vi "endianness test.vi"() -> ()   [LabVIEW 2013, in "Profibus Module tests.lvlib"]
uses:
  Profibus Module tests.lvlib
  execution/profibus slave configuration.ctl
  execution/profibus mapping configuration.ctl
  <vilib>/NI/Tag Bus/tag/Data Type.ctl
  configuration/Profibus Module configuration.lvclass
  configuration/endianness setting.ctl
  channel/Profibus channel.lvclass
  <vilib>/NI/Tag Bus Module Framework/channel/channel classification.ctl
  channel/Profibus channel.lvclass/Profibus channel.ctl
  <vilib>/NI/Tag Bus Module Framework/channel/TBM channel.lvclass/TBM channel.ctl
  <vilib>/NI/Tag Bus/tag/tag descriptor.lvclass/tag descriptor.ctl
  configuration/Profibus Module configuration.lvclass/Profibus Module configuration.ctl
  channel/Write slave.vi
  channel/Write byte.vi
  <vilib>/NI/Tag Bus Module Framework/channel/Write channel classification.vi
  <vilib>/NI/Tag Bus/tag/write data type.vi
  <vilib>/NI/Tag Bus/tag/write tag name.vi
  <vilib>/NI/Tag Bus/table/data polymorphs/write one/write U8.vi
  <vilib>/NI/Tag Bus/table/data polymorphs/write one/write U16.vi
  <vilib>/NI/Tag Bus/table/data polymorphs/write one/write U32.vi
  configuration/Write byte orders.vi
  configuration/Read profibus channels.vi
  execution/calculate last byte.vi
  <vilib>/NI/Tag Bus/tag/read tag name.vi
  <vilib>/NI/Tag Bus/tag/read data type.vi
  <vilib>/NI/Tag Bus Module Framework/channel/Read channel classification.vi
  channel/Read slave.vi
  channel/Read byte.vi
  channel/Read bit.vi
  configuration/Read byte orders.vi
  execution/set endianness.vi
  <vilib>/NI/Tag Bus/dictionary/locate tag.vi
  execution/slave not available error.vi
  execution/data out of range.vi
  <vilib>/NI/Tag Bus/dictionary/data dictionary.lvclass
  <vilib>/NI/Tag Bus Module Framework/channel/TBM channel.lvclass
  <vilib>/NI/Tag Bus Module Framework/runtime/TBM module execution interface.lvclass
  execution/Profibus Module runtime.lvclass
  <vilib>/NI/Tag Bus Module Framework/root configuration/TBM configuration.lvclass
  <vilib>/NI/Tag Bus/tag/tag descriptor.lvclass
  <vilib>/NI/Tag Bus/table/data table.lvlib
panel:
  out "in":cluster{"U32":u32, "U16":u16, "U8":u8}[](array[cluster])
  out "16b":u16
  out "16l":u16
  out "32b":u32
  out "32l":u32
  out "u32b":u8[](array[numeric])
  out "u16b":u8[](array[numeric])
  out "out":u8[][](array[numeric])
  out "outputs":T1[](array[typedef])
  out "inputs":T1[](array[typedef])
  out "error out":errorcluster
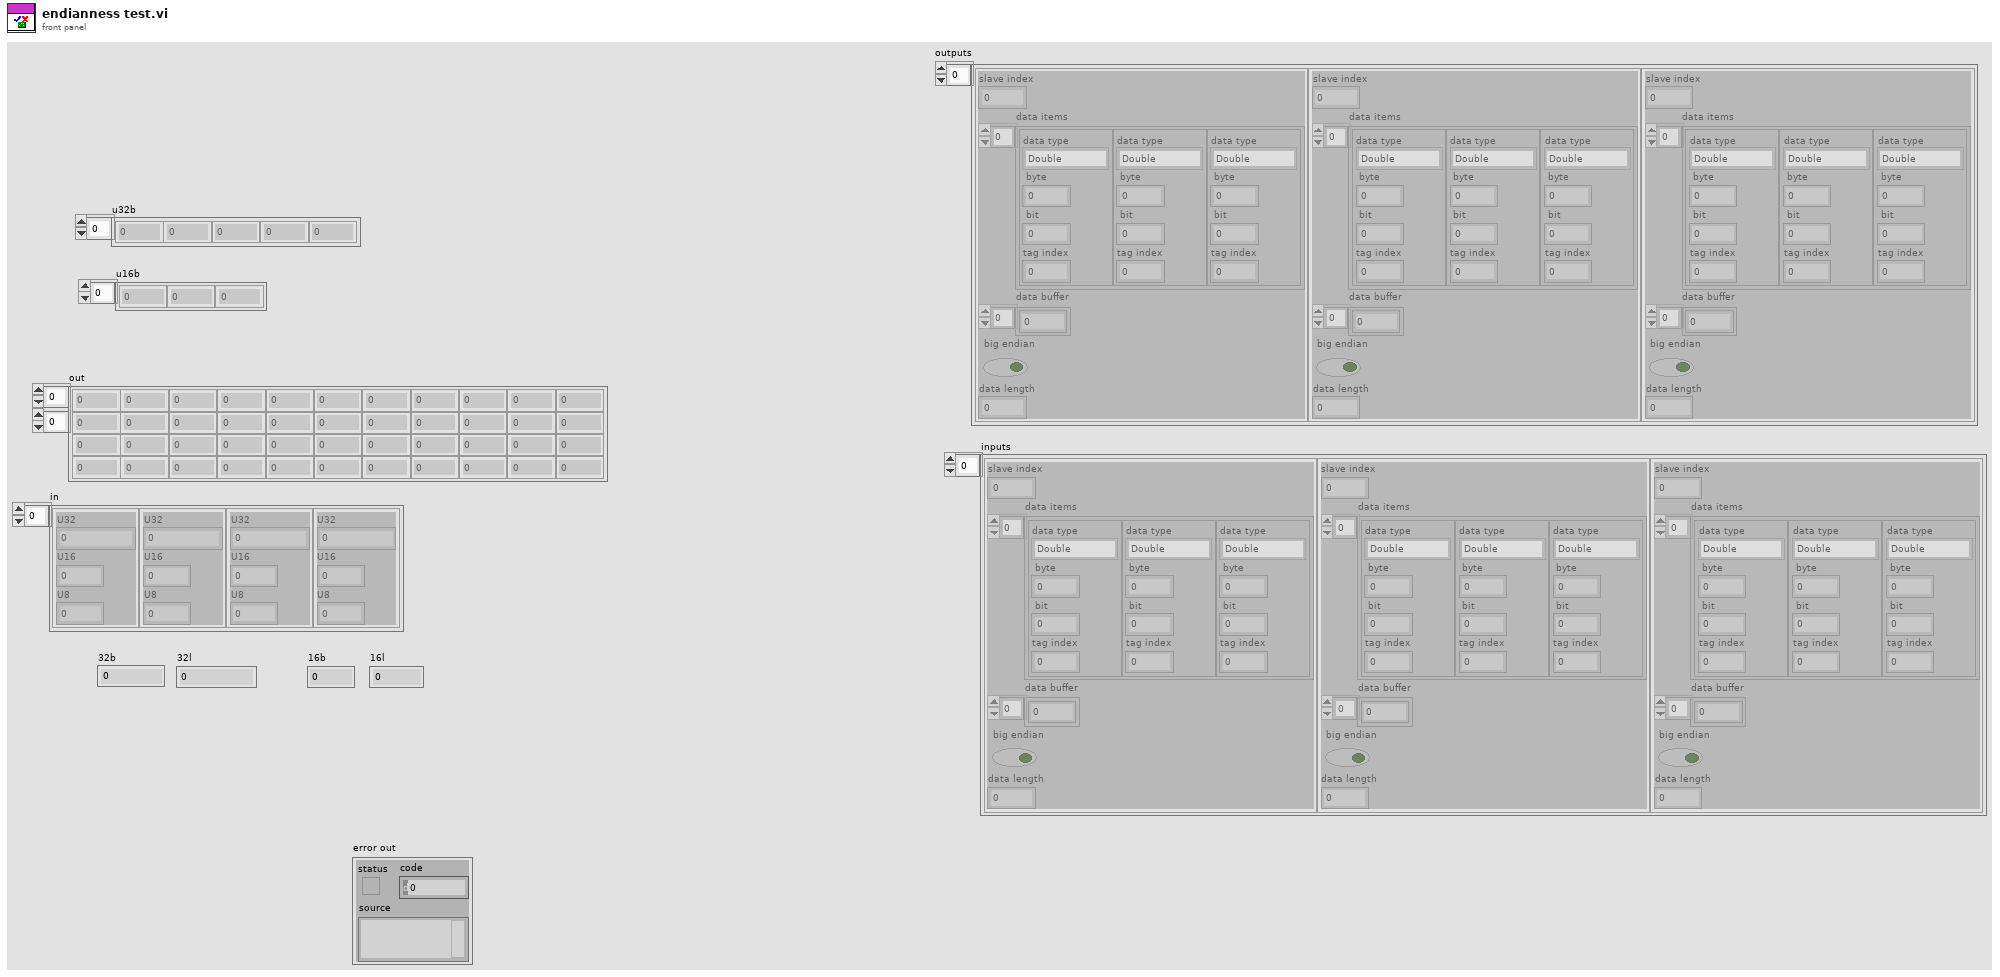
[diagram p1: front panel]
types:
  T1 = typedef "Profibus Module runtime.lvclass/profibus slave configuration.ctl" = cluster{"slave index":i8, "data items":T2[], "data buffer":u8[], "big endian":bool, "data length":i32}
  T2 = typedef "Profibus Module runtime.lvclass/profibus mapping configuration.ctl" = cluster{"data type":T3, " byte":i32, " bit":i32, "tag index":i32}
  T3 = typedef "tag bus.lvlib/tag descriptor.lvclass/Data Type.ctl" = enum16{"Double", "Single", "I64", "I32", "I16", "I8", "U64", "U32", "U16", "U8", "Boolean", "String", "Array of Double", "Array of Single", "Array of I64", "Array of I32", "Array of I16", "Array of I8", "Array of U64", "Array of U32", "Array of U16", "Array of U8", "Array of Boolean", "Array of String"}
  T4 = typedef "TBM channel.lvclass/channel classification.ctl" = enum16{"input data", "output data", "processing parameter", "processing result"}
  T5 = cluster{"Address":i8, "Input Length":u8, "Output Length":u8}[]
  T6 = typedef "Profibus Module configuration.lvclass/endianness setting.ctl" = cluster{"slave":i8, "big endian":bool}
  T7 = typedef "TBM channel.lvclass/data tables.ctl" = cluster{"input data":T8, "processing parameter":T8, "processing result":T8, "output data":T8}
  T8 = typedef "tag bus.lvlib/dictionary table pair.ctl" = cluster{"data dictionary":refnum<class "data dictionary.lvclass">, "data table":T9}
  T9 = typedef "tag bus.lvlib/data table.lvlib/data table.ctl" = cluster{"Double":dbl[], "Single":sgl[], "I64":i64[], "I32":i32[], "I16":i16[], "I8":i8[], "U64":u64[], "U32":u32[], "U16":u16[], "U8":u8[], "Boolean":bool[], "String":string[], "Array of Double":cluster{"DBL Array":dbl[]}[], "Array of Single":cluster{"SGL Array":sgl[]}[], "Array of I64":cluster{"I64 Array":i64[]}[], "Array of I32":cluster{"I32 Array":i32[]}[], "Array of I16":cluster{"I16 Array":i16[]}[], "Array of I8":cluster{"I8 Array":i8[]}[], "Array of U64":cluster{"U64 Array":u64[]}[], "Array of U32":cluster{"U32 Array":u32[]}[], "Array of U16":cluster{"U16 Array":u16[]}[], "Array of U8":cluster{"U8 Array":u8[]}[], "Array of Boolean":cluster{"Boolean Array":bool[]}[], "Array of String":cluster{"String Array":string[]}[]}
  T10 = typedef "TBM module execution interface.lvclass/execution settings.ctl" = cluster{"reads inputs":bool, "processes data":bool, "writes outputs":bool}
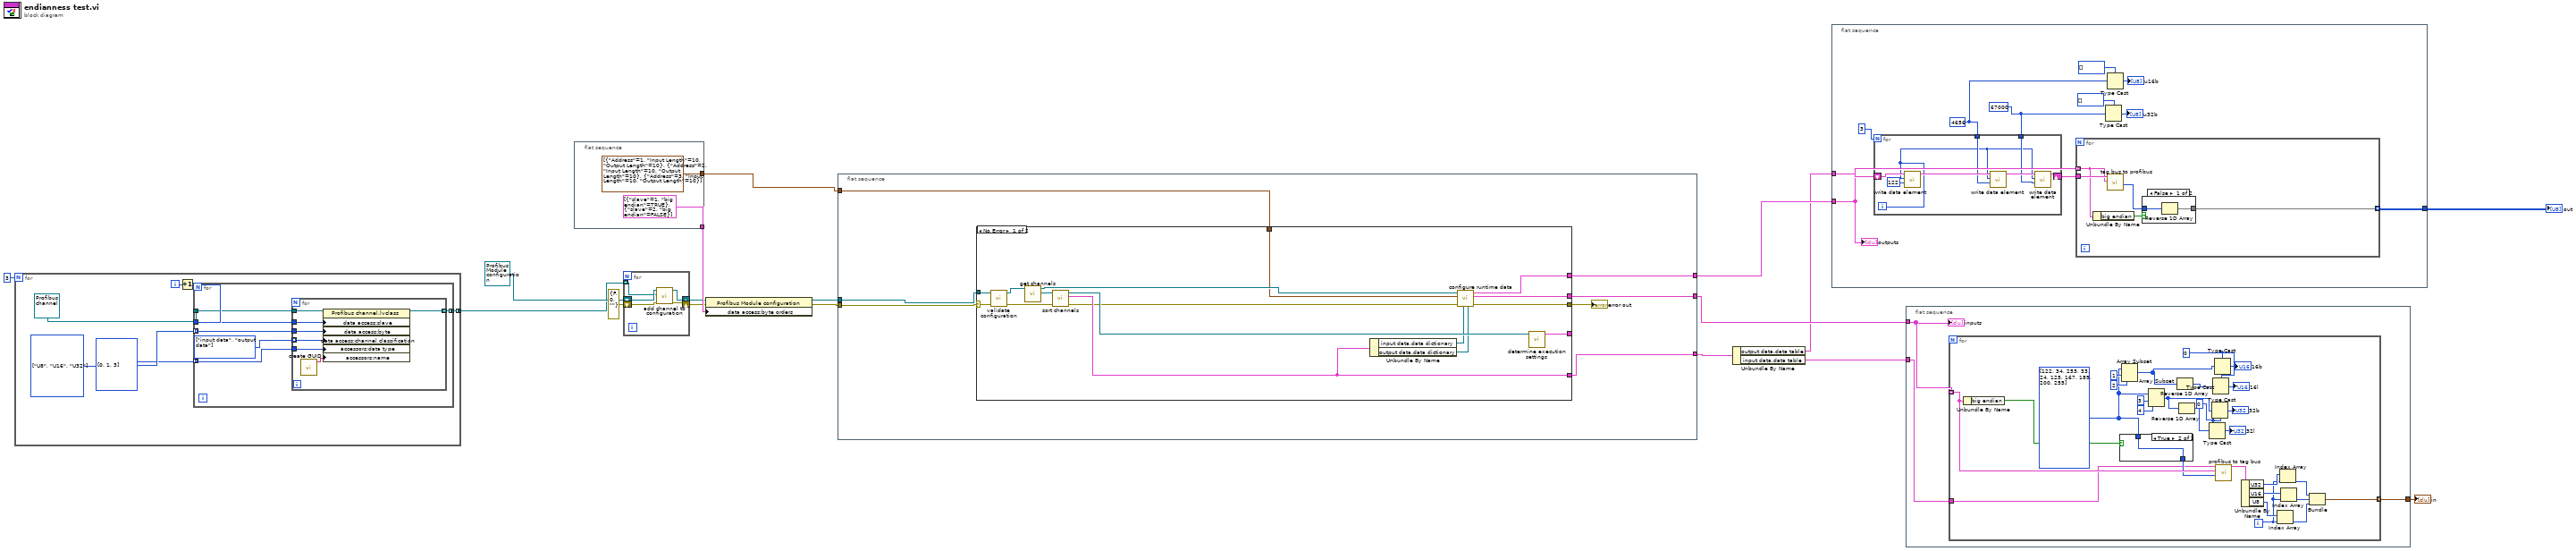
[diagram p0: block diagram]
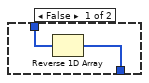
[diagram p2: hidden frame]
diagram:
  n1 = for {
    N: 3 -> [_]
    tunnel: [w22] -> w9 mode=concatenating
    i -> [w21]
    w18 = T3[] [enum."U8", enum."U16", enum."U32"] items=["Double", "Single", "I64", "I32", "I16", "I8", "U64", "U32", "U16", "U8", "Boolean", "String", "Array of Double", "Array of Single", "Array of I64", "Array of I32", "Array of I16", "Array of I8", "Array of U64", "Array of U32", "Array of U16", "Array of U8", "Array of Boolean", "Array of String"]
    n2 = Increment(x=w21) -> (x+1=w20:i32)
    n3 = for {
      tunnel: refnum<class "Profibus channel.lvclass"> refnum ("Profibus channel.lvclass") -> [w29]
      tunnel: [w28] -> w22 mode=concatenating
      tunnel: w20 -> [w27]
      tunnel: i32[] [0, 1, 3] -> [w25] mode=indexing
      tunnel: w18 -> [w24] mode=indexing
      w26 = T4[] [enum."input data", enum."output data"] items=["input data", "output data", "processing parameter", "processing result"]
      n4 = for {
        tunnel: w29 -> [w36]
        tunnel: [w35] -> w28 mode=indexing
        tunnel: w27 -> [w34]
        tunnel: w26 -> [w32] mode=indexing
        tunnel: w25 -> [w31]
        tunnel: w24 -> [w30]
        n5 = call <vilib>:"create GUID.vi"() -> ("uuid"=w33:string)  [unwired: 11 in]
        n6 = property class="Profibus channel.lvclass"(reference=w36, "data access:slave"=w34, "data access:byte"=w31, "data access:channel classification"=w32, "accessors:data type"=w30, "accessors:name"=w33) -> (reference out=w35:refnum<class "Profibus channel.lvclass">)  [unwired: 1 in, 1 out]
      }
    }
  }
  n7 = flat-sequence {
    tunnel: [T6[] [{"slave"=1, "big endian"=TRUE}, {"slave"=2, "big endian"=FALSE}] ("byte orders")] -> w17
    tunnel: [T5 [{"Address"=1, "Input Length"=10, "Output Length"=10}, {"Address"=2, "Input Length"=10, "Output Length"=10}, {"Address"=3, "Input Length"=10, "Output Length"=10}] ("Slave Info List")] -> w16
    frame #0 {
    }
  }
  n8 = for {
    shift-right: [w43] -> w13
    shift-left: refnum<class "Profibus Module configuration.lvclass"> refnum ("Synchronous module configuration") -> [w41]
    shift-right: [w42] -> w12
    shift-left: errorcluster {"status"=FALSE, "code"=0, "source"=""} ("error out") -> [w40]
    tunnel: w9 -> [w39] mode=indexing
    n9 = call "add channel to configuration.vi"("error in"=w40, "TBM channel in"=w39, "Profibus Module configuration in"=w41) -> ("error out"=w42:errorcluster, "Profibus Module configuration out"=w43:refnum<class "Profibus Module configuration.lvclass">)  [unwired: 7 in]
  }
  n10 = property class="Profibus Module configuration"(reference=w13, error in=w12, "data access:byte orders"=w17) -> (reference out=w15:refnum<class "Profibus Module configuration.lvclass">, error out=w14:errorcluster)
  n11 = flat-sequence {
    tunnel: w16 -> [w47]
    tunnel: w15 -> [w49]
    tunnel: w14 -> [w48]
    tunnel: [w46] -> w7
    tunnel: [w45] -> w6
    tunnel: [w44] -> w5
    frame #0 {
      n12 = case shown="No Error" w48 {
        selector: w48 -> [w63 w67]
        tunnel: w49 -> [w62 _]
        tunnel: [w59 w67] -> w50
        tunnel: [w58 _] -> w44
        tunnel: [w66 _] -> _
        tunnel: w47 -> [w53 _]
        tunnel: [w52 _] -> w46
        tunnel: [w51 _] -> w45
        frame No Error {
          n13 = call-dynamic "validate configuration.vi"("error in"=w63, "Profibus Module configuration in"=w62) -> ("error out"=w64:errorcluster, "Profibus Module configuration out"=w61:refnum<class "Profibus Module configuration.lvclass">)  [unwired: 8 in]
          n14 = call-dynamic "get channels.vi"("Profibus Module configuration in"=w61) -> ("channels"=w60:refnum<class "TBM channel.lvclass">[], "Profibus Module configuration out"=w55:refnum<class "Profibus Module configuration.lvclass">)  [unwired: 9 in]
          n15 = call <vilib>:"sort channels.vi"("error in"=w64, "channels in"=w60) -> ("error out"=w54:errorcluster, "data allocations"=w58:T7, "channels out"=w65:refnum<class "TBM channel.lvclass">[])  [unwired: 7 in]
          n16 = Unbundle By Name(w58) -> ("input data.data dictionary"=w56:refnum<class "data dictionary.lvclass">, "output data.data dictionary"=w57:refnum<class "data dictionary.lvclass">)
          n17 = call "configure runtime data.vi"("output dictionary"=w57, "input dictionary"=w56, "error in"=w54, "Slave Info List"=w53, "Profibus Module configuration in"=w55) -> ("error out"=w59:errorcluster, "inputs"=w51:T1[], "outputs"=w52:T1[])  [unwired: 4 in]
          n18 = call <vilib>:"determine execution settings.vi"("channels"=w65) -> ("execution settings"=w66:T10)  [unwired: 10 in]
        }
        frame Error {
        }
      }
      "error out" <- w50
    }
  }
  n19 = Unbundle By Name(w5) -> ("output data.data table"=w4:T9, "input data.data table"=w3:T9)
  n20 = flat-sequence {
    tunnel: w7 -> [w77]
    tunnel: w4 -> [w78]
    tunnel: [w76] -> w2
    frame #0 {
      w68 = u16 4656 ("value")
      w69 = u32 67000 ("value")
      n21 = for {
        N: 3 ("index") -> [_]
        tunnel: w69 -> [w81]
        tunnel: w68 -> [w80]
        shift-right: [w84] -> w75
        shift-left: w78 -> [w86]
        i -> [w79]
        n22 = call-poly <vilib>:"write data element.vi"("value"=u8 122, "index"=w79, "data table in"=w86) -> ("data table out"=w83:T9)  [unwired: 8 in]
        n23 = call-poly <vilib>:"write data element.vi"("value"=w80, "index"=w79, "data table in"=w83) -> ("data table out"=w85:T9)  [unwired: 8 in]
        n24 = call-poly <vilib>:"write data element.vi"("value"=w81, "index"=w79, "data table in"=w85) -> ("data table out"=w84:T9)  [unwired: 8 in]
      }
      n25 = for {
        tunnel: w77 -> [w88] mode=indexing
        tunnel: [w87] -> w76 mode=indexing
        tunnel: w75 -> [w91]
        n26 = Unbundle By Name(w88) -> ("big endian"=w90:bool)
        n27 = call "tag bus to profibus.vi"("slave configuration"=w88, "data table in in"=w91) -> ("Data"=w89:u8[])  [unwired: 7 in, 2 out]
        n28 = case shown="False" w90 {
          tunnel: [w92 w94] -> w87
          tunnel: w89 -> [w93 w94]
          frame False {
            n29 = Reverse 1D Array(array=w93) -> (reversed array=w92:u8[])
          }
          frame True {
          }
        }
      }
      n30 = Type Cast(type=u8[] [] ("Data"), x=w69) -> (*(type *) &x=→"u32b":u8[])
      n31 = Type Cast(type=u8[] [] ("Data"), x=w68) -> (*(type *) &x=→"u16b":u8[])
      "outputs" <- w77
    }
  }
  n32 = flat-sequence {
    tunnel: w6 -> [w96]
    tunnel: w3 -> [w97]
    tunnel: [w95] -> w1
    frame #0 {
      n33 = for {
        tunnel: w96 -> [w125] mode=indexing
        tunnel: w97 -> [w99]
        tunnel: [w100] -> w95 mode=indexing
        i -> [w98]
        w112 = u16 0 ("value")
        w113 = u32 0 ("value")
        w118 = u8[] [122, 34, 253, 33, 24, 125, 167, 189, 200, 255] ("Data out")
        n34 = Unbundle By Name(w125) -> ("big endian"=w124:bool)
        n35 = case shown="True" w124 {
          tunnel: [w126 w128] -> w123
          tunnel: w118 -> [w127 w128]
          frame False {
            n36 = Reverse 1D Array(array=w127) -> (reversed array=w126:u8[])
          }
          frame True {
          }
        }
        n37 = Array Subset(array=w118, index=1, length=2) -> (w117:u8[])
        n38 = Array Subset(array=w118, index=3, length=4) -> (w115:u8[])
        n39 = Reverse 1D Array(array=w117) -> (reversed array=w116:u8[])
        n40 = Reverse 1D Array(array=w115) -> (reversed array=w114:u8[])
        n41 = Type Cast(type=w113, x=w114) -> (*(type *) &x=→"32l":u32)
        n42 = Type Cast(type=w113, x=w115) -> (*(type *) &x=→"32b":u32)
        n43 = Type Cast(type=w112, x=w116) -> (*(type *) &x=→"16l":u16)
        n44 = Type Cast(type=w112, x=w117) -> (*(type *) &x=→"16b":u16)
        n45 = call "profibus to tag bus.vi"("Data in"=w123, "slave configuration"=w125, "data table in"=w99) -> ("data table out"=w107:T9)  [unwired: 8 in]
        n46 = Unbundle By Name(w107) -> ("U32"=w106:u32[], "U16"=w105:u16[], "U8"=w104:u8[])
        n47 = Index Array(array=w104, index=w98) -> (element=w101:u8)
        n48 = Index Array(array=w106, index=w98) -> (element=w103:u32)
        n49 = Index Array(array=w105, index=w98) -> (element=w102:u16)
        n50 = Bundle("U32"=w103, "U16"=w102, "U8"=w101) -> (w100:cluster{"U32":u32, "U16":u16, "U8":u8})  [unwired: 1 in]
      }
      "inputs" <- w96
    }
  }
  "out" <- w2
  "in" <- w1
